vi "Calculate Averaged Resistance.vi"(11 "SMU Measurements":T1) -> (1 "Averaged Resistance":dbl[][](array[numeric]), 2 "Calculated Negative Resistance":dbl[][](array[numeric]), 3 "Calculated Positive Resistance":dbl[][](array[numeric]))   [LabVIEW 2013]
uses:
  Controls/SMU Measurements.ctl
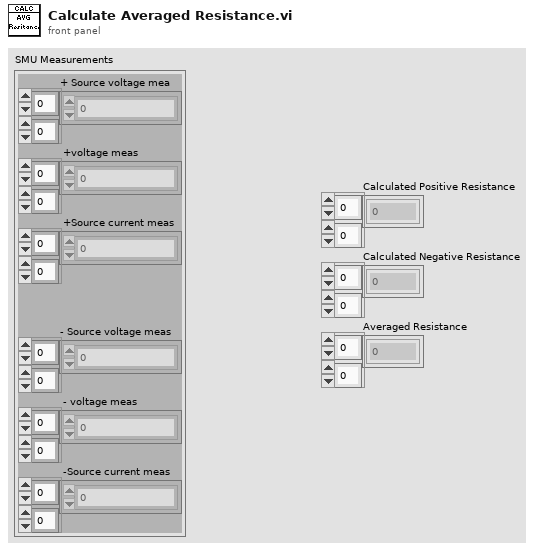
[diagram p1: front panel]
types:
  T1 = typedef "SMU Measurements.ctl" = cluster{"+ Source voltage mea":dbl[][], " +voltage meas":dbl[][], "- Source voltage meas":dbl[][], " - voltage meas":dbl[][], " +Source current meas":dbl[][], " -Source current meas":dbl[][]}
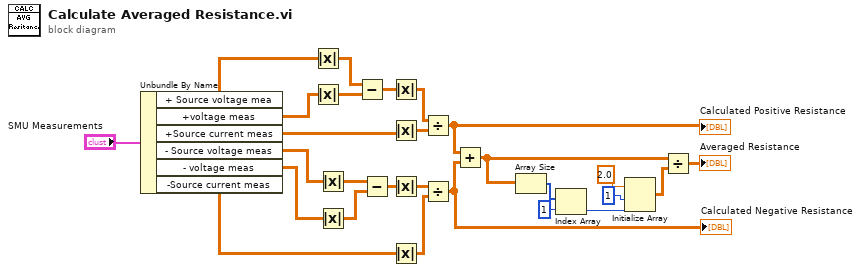
[diagram p0: block diagram]
diagram:
  n1 = Unbundle By Name("SMU Measurements") -> ("+ Source voltage mea"=w6:dbl[][], "+voltage meas"=w5:dbl[][], "+Source current meas"=w4:dbl[][], "- Source voltage meas"=w3:dbl[][], "- voltage meas"=w2:dbl[][], "-Source current meas"=w1:dbl[][])
  n2 = Absolute Value(x=w6) -> (abs(x)=w27:dbl[][])
  n3 = Absolute Value(x=w5) -> (abs(x)=w26:dbl[][])
  n4 = Absolute Value(x=w3) -> (abs(x)=w24:dbl[][])
  n5 = Absolute Value(x=w2) -> (abs(x)=w23:dbl[][])
  n6 = Subtract(x=w27, y=w26) -> (x-y=w25:dbl[][])
  n7 = Subtract(x=w24, y=w23) -> (x-y=w22:dbl[][])
  n8 = Absolute Value(x=w25) -> (abs(x)=w21:dbl[][])
  n9 = Absolute Value(x=w4) -> (abs(x)=w20:dbl[][])
  n10 = Absolute Value(x=w22) -> (abs(x)=w19:dbl[][])
  n11 = Absolute Value(x=w1) -> (abs(x)=w18:dbl[][])
  n12 = Divide(x=w21, y=w20) -> (x/y=w17:dbl[][])
  "Calculated Positive Resistance" <- w17
  n13 = Divide(x=w19, y=w18) -> (x/y=w16:dbl[][])
  "Calculated Negative Resistance" <- w16
  n14 = Add(x=w17, y=w16) -> (x+y=w9:dbl[][])
  n15 = Array Size(array=w9) -> (size(s)=w13:i32[])
  n16 = Index Array(array=w13, index=1) -> (element=w11:i32)
  n17 = Initialize Array(2.0 ("element"), 1 ("dimension size"), w11) -> (w8:dbl[][])
  n18 = Divide(x=w9, y=w8) -> (x/y=→"Averaged Resistance":dbl[][])
